vi "DB5000.W读取.vi"(0 "gInitialSIEMENSS7 In":refnum<k24>, 1 "地址数组":string[](array[string])=["DB5000.228"], 5 "error in (no error)":errorcluster caption="错误输入（无错误）") -> (14 "gInitialSIEMENSS7 Out":refnum<k24>, 15 "IsSuccess":bool, 16 "Content":u16, 18 "Message":string, 19 "error out":errorcluster caption="错误输出")   [LabVIEW 2017]
panel:
  in  "一致性检测结果 2":u16
  out "数值":i32
  out "数组 2":string[](array[string])
  # "DB5000,W228"
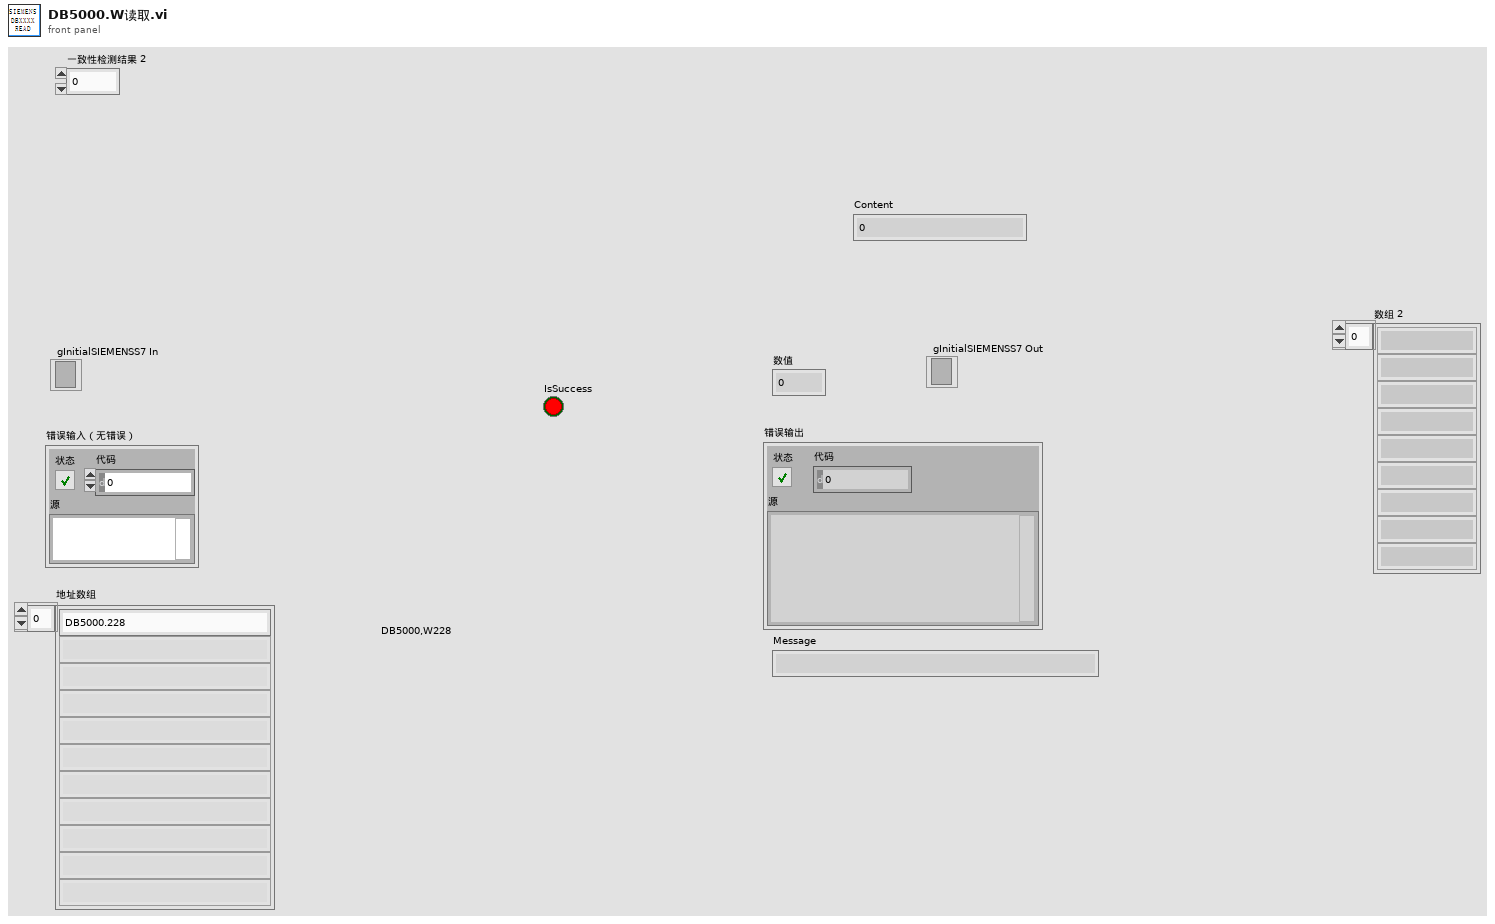
[diagram p1: front panel]
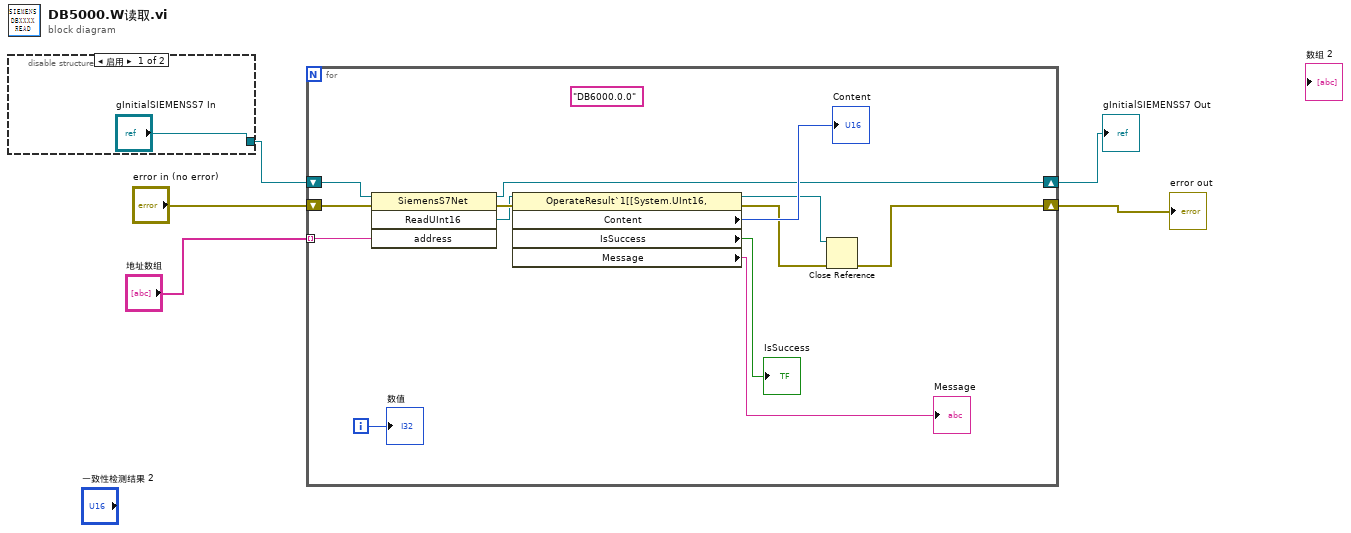
[diagram p0: block diagram]
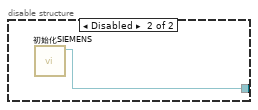
[diagram p2: hidden frame]
diagram:
  n1 = disable-structure shown="启用" {
    disable-tunnel: ["gInitialSIEMENSS7 In" w7] -> w2
    frame Enabled {
    }
    frame Disabled {
      n2 = call "初始化SIEMENS.vi"() -> ("gInitialSIEMENSS7"=w7:refnum<k24>)  [unwired: 9 in, 2 out]
    }
  }
  n3 = for {
    tunnel: "地址数组" -> [w12] mode=indexing
    shift-right: [w8] -> w3
    shift-left: "error in (no error)" -> [w20]
    shift-right: [w11] -> w4
    shift-left: w2 -> [w13]
    i -> [w15]
    (unwired) "DB6000.0.0" ("address")
    n4 = invoke class="SiemensS7Net" method="ReadUInt16"(reference=w13, error in=w20, "address"=w12) -> (reference out=w11:refnum<k24>, error out=w19:errorcluster, "ReadUInt16"=w18:refnum<k24>)  [unwired: 1 in, 1 out]
    n5 = property class="OperateResult`1[[System.UInt16,"(reference=w18, error in=w19) -> (reference out=w10:refnum<k24>, error out=w9:errorcluster, "Content"=→"Content":u16, "IsSuccess"=→"IsSuccess":bool, "Message"=→"Message":string)
    n6 = Close Reference(reference=w10, error in (no error)=w9) -> (error out=w8:errorcluster)
    "数值" <- w15
  }
  "gInitialSIEMENSS7 Out" <- w4
  "error out" <- w3
